vi "data_prepare.vi"(11 "base path":path) -> (3 "all rows":dbl[][](array[numeric]))   [LabVIEW 2022 SP3]
uses:
  <vilib>/Utility/file.llb/Read Delimited Spreadsheet (DBL).vi
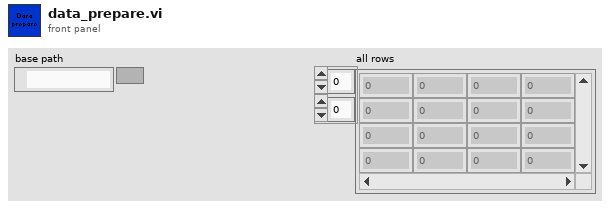
[diagram p1: front panel]
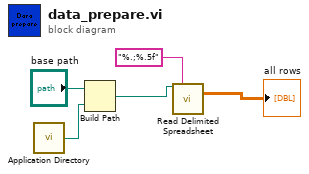
[diagram p0: block diagram]
diagram:
  n1 = call <vilib>:"Application Directory.vi"() -> ("Application Directory"=w4:path)
  n2 = Build Path(base path="base path", name or relative path=w4) -> (appended path=w3:path)
  n3 = call-poly <vilib>:"Read Delimited Spreadsheet.vi"("file path (dialog if empty)"=w3, "format (%.3f)"="%.;%.5f") -> ("all rows"=→"all rows":dbl[][])  [unwired: 8 in, 5 out]
